vi "Monitor Transmit and Receive Messages.vi"() -> ()   [LabVIEW 2019]
doc: "This program opens the specified card, finds the first compatible core, builds a transmit schedule using transmit interval information, and creates filters for two receive messages. It also enables the Sequential Monitor to record transmitted and received messages."
uses:
  <instrlib>/BTI429Lib/Public/Controls/429 Record.ctl
  <instrlib>/BTICardLib/Private/Initialize By Card Number and Core Number.vi
  <instrlib>/BTICardLib/Private/Configure Core From Bin.vi
  <instrlib>/BTI429Lib/Private/Tx/Configure/Configure Tx Channel From Bin.vi
  <instrlib>/BTI429Lib/Private/Rx/Configure/Configure Rx Channel From Bin.vi
  <instrlib>/BTI429Lib/Private/Core/Action-Status/Start All Channels.vi
  <instrlib>/BTI429Lib/Private/Core/Action-Status/Stop All Channels.vi
  <instrlib>/BTICardLib/BTICardLV.lvlib
  <instrlib>/BTI429Lib/BTI429LV.lvlib
panel:
  out "rx channel number":i32
  out "tx channel number":i32=16
  out "core number":i32
  in  "Rx Channel Configuration File":string="../../ballard/Rx Channel Config.FINF"
  in  "Tx Channel Configuration File":string="../../ballard/Tx Channel Config.FINF"
  out "record out":T1 {"type" format="%04x"; "timestamp" format="%08x"; "msgact" format="%04x"; "data" format="%08x"; "timestamph" format="%08x"}
  in  "Core Configuration File":string="../../ballard/Core Config.FINF"
  in  "stop":bool
  out "error out":errorcluster={"status"=TRUE, "code"=403003, "source"="BTICardLV.lvlib:Error Converter (ErrCode or Status).vi<ERR>\n403003: Failed to open the file [/home/lvuser/natinst/LabVIEW Data/Core Config.FINF] (When calling LabVIEW Library function BTICardLV_ConfigureCoreFromBin, encountered error 403003=ERRTYPE_CONFIG Error occurred parsing the configuration file (LabVIEW Library) with internal error -34=ERR_NOCONFIG The card has not been properly configured (BTICard))\n\n\n<b>Complete call chain:</b>\n     BTICardLV.lvlib:Error Converter (ErrCode or Status).vi\n     BTICardLV.lvlib:Configure Core From Bin.vi\n     Monitor Transmit and Receive Messages.vi"}
  in  "Card Number":i32
  # "LabVIEW RT"
  # "ARINC 429: Monitor Transmit and Receive Messages"
  # "©2016 Astronics Ballard Technology"
  # "This program opens the specified card, finds the first compatible core, builds a transmit schedule using transmit interval information, and creates filters for two receive messages.  It also enables the Sequential Monitor to record transmitted and received messages."
  # "!!For LinuxRT, base path is /home/lvuser/natinst/LabVIEW Data"
  # "LabVIEW RT can parse both XML and Binary (FINF or Fast Infoset) configuration files. While the Binary files are non-human readable, they can be loaded and parsed much more quickly than XML and are also smaller. These can also be used in LabVIEW for Windows.\n\nLabVIEW RT examples use the Binary configuration file and the corollary \"Configure From Bin\" VIs. Using the XML is as simple as switching the polymorphic configuration VI from \"Binary\" to \"XML\" and changing the Configuration Filename above."
  # "Always Stop the card\nand Close the card when\ndone. Otherwise, the hardware\ncontinues to operate."
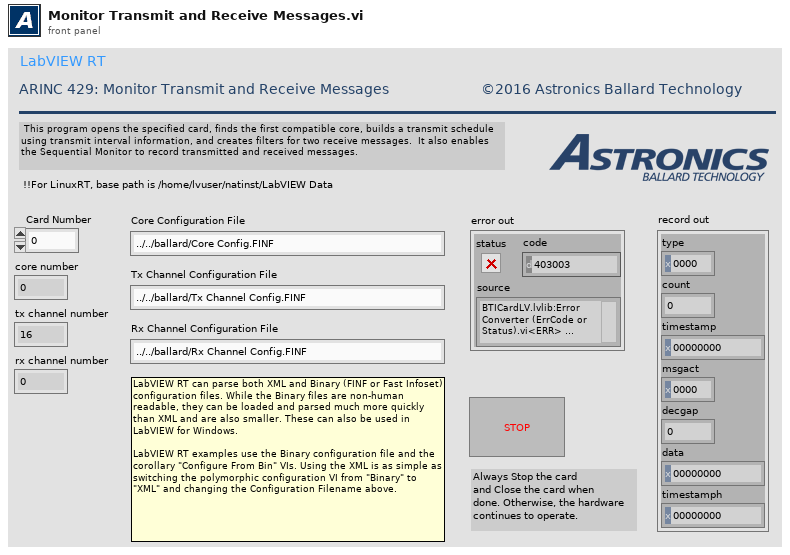
[diagram p1: front panel]
types:
  T1 = typedef "BTI429LV.lvlib/429 Record.ctl" = cluster{"type":u16, "count":u16, "timestamp":u32, "msgact":u16, "decgap":u16, "data":u32, "timestamph":u32}
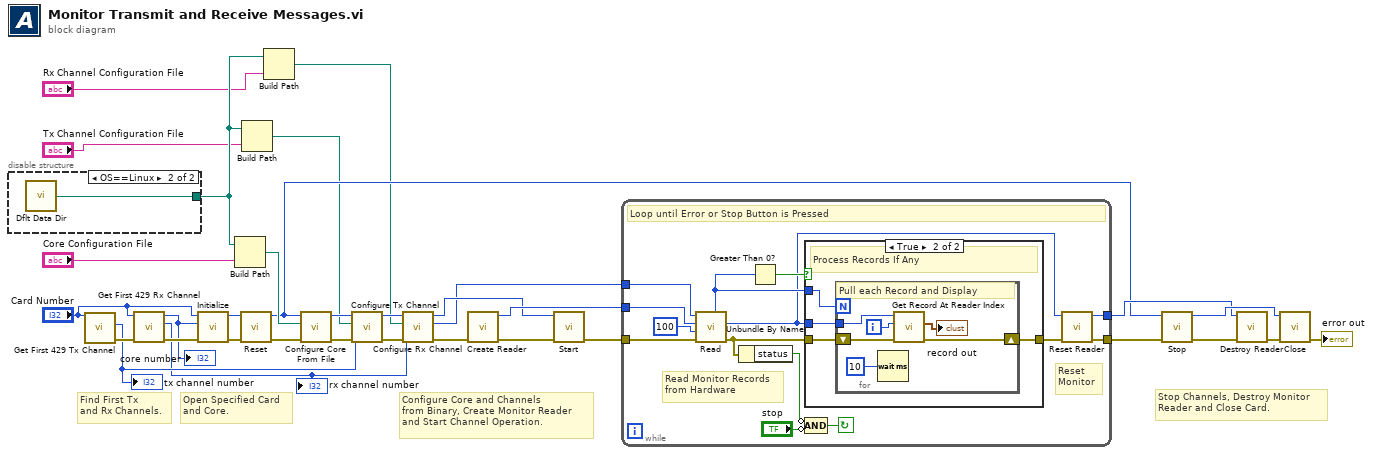
[diagram p0: block diagram]
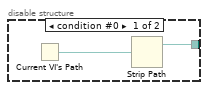
[diagram p2: hidden frame]
diagram:
  # "Find First Tx \nand Rx Channels."
  # "Stop Channels, Destroy Monitor\nReader and Close Card."
  # "Configure Core and Channels \nfrom Binary, Create Monitor Reader \nand Start Channel Operation."
  # "Open Specified Card\nand Core."
  n1 = disable-structure shown="OS==Linux" {
    disable-tunnel: [w34 w36] -> w18
    frame condition #0 {
      n2 = Current VI's Path() -> (path=w35:path)
      n3 = Strip Path(path=w35) -> (stripped path=w34:path)  [unwired: 1 out]
    }
    frame condition #1 (active) {
      n4 = call <vilib>:"Dflt Data Dir.vi"() -> ("App:Default Data Directory"=w36:path)
    }
  }
  n5 = call "Get First 429 Tx Channel.vi"("Card Number"="Card Number") -> ("error out"=w6:errorcluster, "Channel Number"=w3:i32)  [unwired: 8 in, 1 out]
  "tx channel number" <- w3
  n6 = call "Get First 429 Rx Channel.vi"("error in (no error)"=w6, "Card Number"="Card Number") -> ("error out"=w5:errorcluster, "Channel Number"=w2:i32, "Core Number"=w1:i32)  [unwired: 7 in]
  "core number" <- w1
  "rx channel number" <- w2
  n7 = call-poly <instrlib>:"Initialize.vi"("error in (no error)"=w5, "core number"=w1, "card number"="Card Number") -> ("error out"=w20:errorcluster, "core handle out"=w21:u64)  [unwired: 7 in]
  n8 = Build Path(base path=w18, name or relative path="Core Configuration File") -> (appended path=w29:path)
  n9 = call <instrlib>:"Reset.vi"("error in (no error)"=w20, "core handle in"=w21) -> ("error out"=w22:errorcluster, "core handle out"=w19:u64)  [unwired: 8 in]
  n10 = Build Path(base path=w18, name or relative path="Tx Channel Configuration File") -> (appended path=w9:path)
  n11 = Build Path(base path=w18, name or relative path="Rx Channel Configuration File") -> (appended path=w8:path)
  n12 = call-poly <instrlib>:"Configure Core From File.vi"("error in (no error)"=w22, "configuration file path"=w29, "core handle in"=w19) -> ("error out"=w15:errorcluster, "core handle out"=w12:u64)  [unwired: 7 in]
  n13 = call-poly <instrlib>:"Configure Tx Channel.vi"("error in (no error)"=w15, "channel number in"=w3, "configuration file path"=w9, "core handle in"=w12) -> ("error out"=w14:errorcluster, "core handle out"=w11:u64)  [unwired: 5 in, 1 out]
  n14 = call-poly <instrlib>:"Configure Rx Channel.vi"("error in (no error)"=w14, "channel number in"=w2, "configuration file path"=w8, "core handle in"=w11) -> ("error out"=w13:errorcluster, "channel handle out"=w7:u64, "core handle out"=w10:u64)  [unwired: 5 in]
  n15 = call <instrlib>:"Create Reader.vi"("error in (no error)"=w13) -> ("error out"=w27:errorcluster, "reader handle out"=w30:u64)  [unwired: 9 in]
  n16 = call-poly <instrlib>:"Start.vi"("error in (no error)"=w27, "core handle in"=w10) -> ("error out"=w31:errorcluster)  [unwired: 8 in, 1 out]
  n17 = while {
    tunnel: [w41] -> w32
    tunnel: w30 -> [w47]
    tunnel: w31 -> [w48]
    tunnel: w7 -> [w46]
    tunnel: [w37] -> w23
    stop <- w49 continue-if-true
    # "Reset\nMonitor"
    # "Read Monitor Records\nfrom Hardware"
    # "Loop until Error or Stop Button is Pressed"
    n18 = call <instrlib>:"Read.vi"("error in (no error)"=w48, "max records to read"=100, "reader handle in"=w47, "channel handle in"=w46) -> ("error out"=w39:errorcluster, "reader handle out"=w40:u64, "records read"=w42:i32)  [unwired: 3 in, 2 out]
    n19 = Unbundle By Name(w39) -> ("status"=w50:bool)
    n20 = Greater Than 0?(x=w42) -> (x > 0?=w43:bool)
    n21 = case shown="True" w43 {
      tunnel: w40 -> [_ w55]
      tunnel: w42 -> [_ w54]
      tunnel: w39 -> [w51 w52]
      tunnel: [w51 w53] -> w38
      frame False {
      }
      frame True {
        # "Process Records If Any"
        n22 = for {
          N: w54 -> [_]
          tunnel: w55 -> [w61]
          shift-right: [w60] -> w53
          shift-left: w52 -> [w59]
          i -> [w57]
          # "Pull each Record and Display"
          n23 = Wait (ms)(milliseconds to wait=u32 10) -> ()  [unwired: 1 out]
          n24 = call <instrlib>:"Get Record At Reader Index.vi"("error in (no error)"=w59, "record index"=w57, "reader handle in"=w61) -> ("error out"=w60:errorcluster, "record out"=→"record out":T1)  [unwired: 6 in, 1 out]
        }
      }
    }
    n25 = Compound Arithmetic op=AND(invert w50, invert "stop") -> (w49:bool)
    n26 = call <instrlib>:"Reset Reader.vi"("error in (no error)"=w38, "reader handle in"=w40) -> ("error out"=w41:errorcluster, "reader handle out"=w37:u64)  [unwired: 8 in]
  }
  n27 = call-poly <instrlib>:"Stop.vi"("error in (no error)"=w32, "core handle in"=w19) -> ("error out"=w26:errorcluster, "core handle out"=w24:u64)  [unwired: 8 in]
  n28 = call <instrlib>:"Destroy Reader.vi"("error in (no error)"=w26, "reader handle in"=w23) -> ("error out"=w25:errorcluster)  [unwired: 8 in, 1 out]
  n29 = call <instrlib>:"Close.vi"("error in (no error)"=w25, "core handle in"=w24) -> ("error out"=→"error out":errorcluster)  [unwired: 8 in, 1 out]
